vi "Drive Controller.vi"(8 "error in":errorcluster) -> ()   [LabVIEW 2016]
doc: "This VI executes continuously carrying out the current operation and responding to updates or new operation requests. It will often contain the timing or control code that is difficult to place directly in TeleOp. This VI generally opens all sensors and motors and isolates the rest of the robot code from knowing implementation details of how the operations are carried out."
uses:
  Drive Setpoints.ctl
  Drive Operations.ctl
  <vilib>/Rock Robotics/WPI/SafetyOutput/WPI_SafetyOutputConfigMenu.ctl
  <vilib>/Rock Robotics/SystemInterfaces/DIO/FPGA_DIOPWMChannel.ctl
  Utility/Drive for Distance States.ctl
  <vilib>/Rock Robotics/WPI/RobotDrive/WPI_RobotDriveOpen4MotorWithTalon.vi
panel:
  out "Setpoints":T1(graph)
  out "Current\nCmd":string
  # "Tip: It may be helpful to observe inputs and sensor values.\nYou may also want to display tuning or debugging controls."
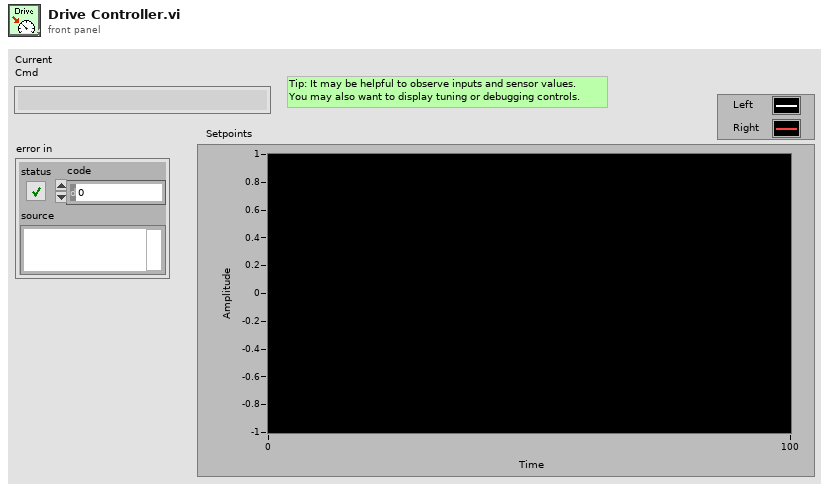
[diagram p1: front panel]
types:
  T1 = cluster{"Left Setpoint":dbl, "Right Setpoint":dbl}
  T2 = typedef "FPGA_DIOPWMChannel.ctl" = enum8{"PWM 0", "PWM 1", "PWM 2", "PWM 3", "PWM 4", "PWM 5", "PWM 6", "PWM 7", "PWM 8", "PWM 9", "PWM MXP 0", "PWM MXP 1", "PWM MXP 2", "PWM MXP 3", "PWM MXP 4", "PWM MXP 5", "PWM MXP 6", "PWM MXP 7", "PWM MXP 8", "PWM MXP 9", "Invalid"}
  T3 = typedef "WPI_SafetyOutputConfigMenu.ctl" = enum16{"Enable", "Disable"}
  T4 = typedef "Drive Setpoints.ctl" = cluster{"Operation":T5, "Left Setpoint":dbl, "Right Setpoint":dbl, "Duration":dbl, "Distance":dbl, "Degrees Rotation":dbl, "Clockwise?":bool}
  T5 = typedef "Drive Operations.ctl" = enum16{"Reserve", "Read Current", "Immediate", "Drive for Time", "Drive for Distance", "Rotate"}
  T6 = typedef "WPI_RobotDriveDevRef.ctl" = cluster{"DevStatus":errorcluster, "Motors[]":T7[], "Square Inputs":bool, "Max Output":dbl}
  T7 = typedef "WPI_MotorControlDeviceRef.ctl" = cluster{"DeviceStatus":errorcluster, "Type":T8, "PWM":cluster{"PWM Channel":T2, "DeadBand":T9}, "CAN":cluster{"Device Number":u8, "SetOutput VI Ref":variant, "GetOutput VI Ref":variant, "Enable VI Ref":variant, "Disable VI Ref":variant, "Data":variant}, "Invert":bool}
  T8 = typedef "WPI_MotorControlType.ctl" = enum16{"PWM", "CAN"}
  T9 = typedef "WPI_PWMDeadband.ctl" = cluster{"Name":string, "maxPositivePwm":i32, "minPositivePwm":i32, "centerPwm":i32, "maxNegativePwm":i32, "minNegativePwm":i32, "angularRange":u16}
  T10 = typedef "Command Status Info.ctl" = cluster{"Name":string, "Status":T11, "notifier out":T12}
  T11 = typedef "Completion Status.ctl" = enum16{"Successful", "Aborted", "Incomplete"}
  T12 = typedef "Completion Notifier.ctl" = refnum<notifier>
  T13 = cluster{"SubSystem Data":T4, cluster{"Start Time (ms)":u32, "Iterations":i32}, cluster{"Command Info":T10, "Description":string, "SubSystem Data":T4, "notifier out":refnum<notifier>, "Subsystem Name":string}}
  T14 = typedef "Drive for Distance States.ctl" = enum16{"Check Distance", "Initialize Distance"}
  T15 = cluster{"SubSystem Data":T4, cluster{"Start Time (ms)":u32, "Iterations":i32}, "Default Command Arguments":cluster{"Command Info":T10, "Description":string, "SubSystem Data":T4, "notifier out":refnum<notifier>, "Subsystem Name":string}}
  T16 = cluster{"Don't move motors while reserved":dbl, "Don't move motors while reserved":dbl}
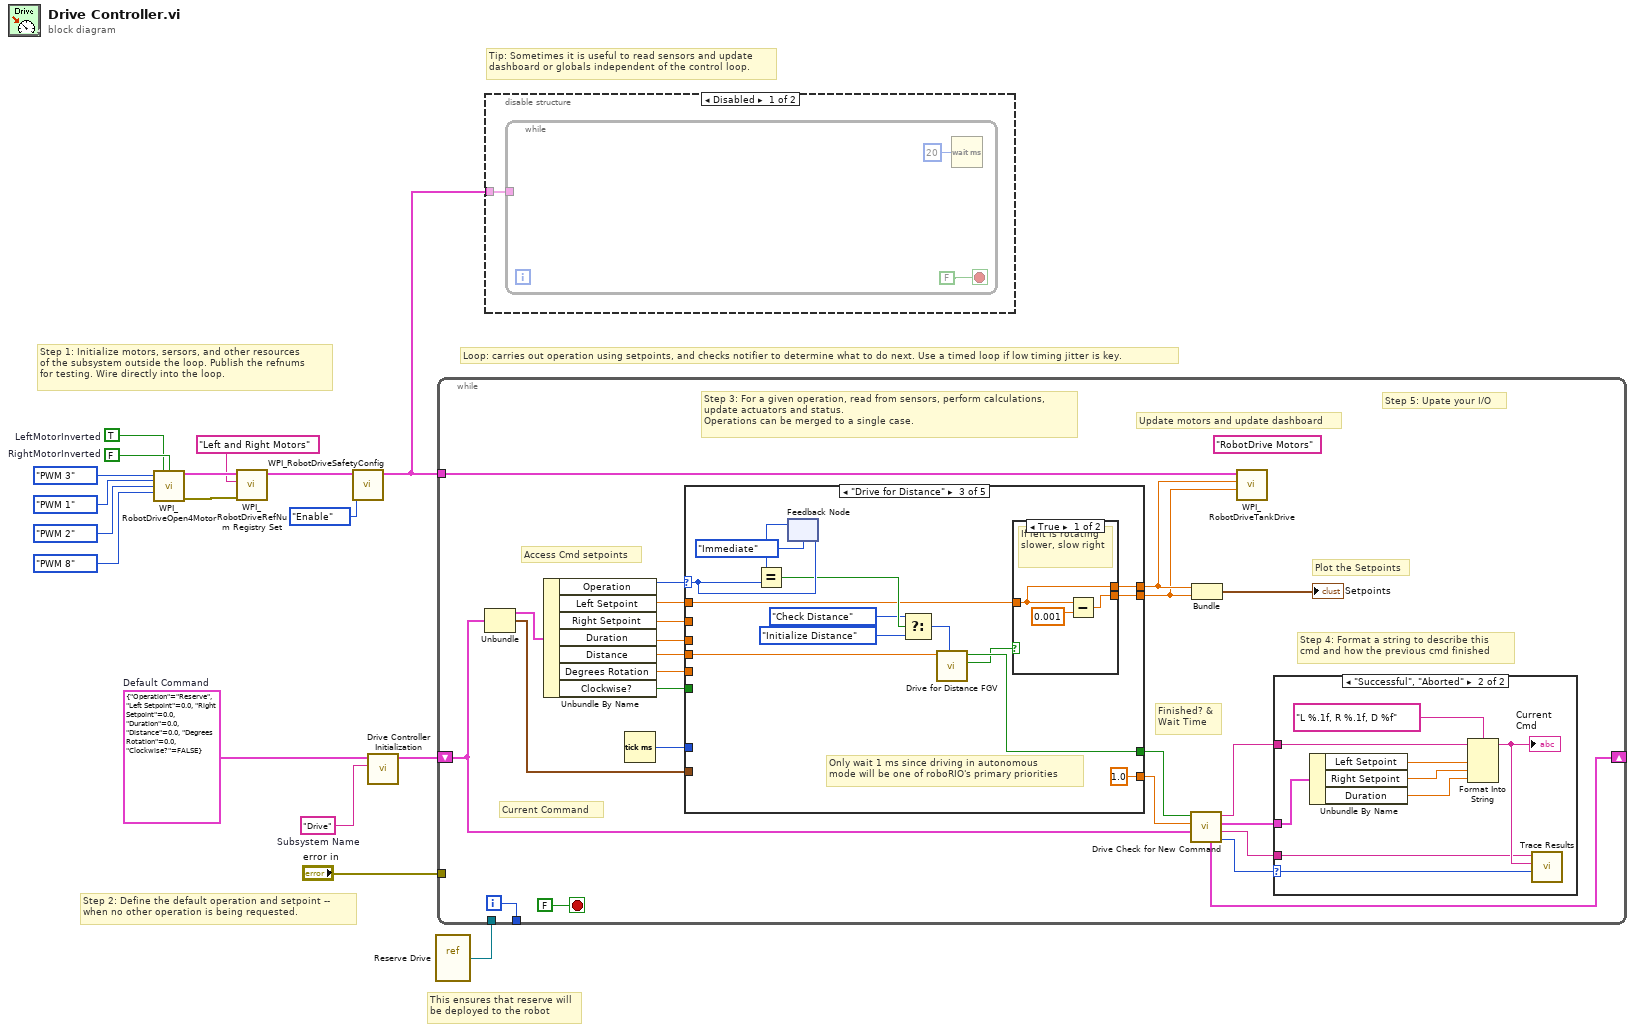
[diagram p0: block diagram]
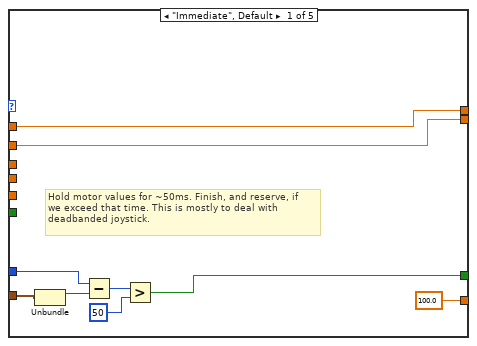
[diagram p4: hidden frame]
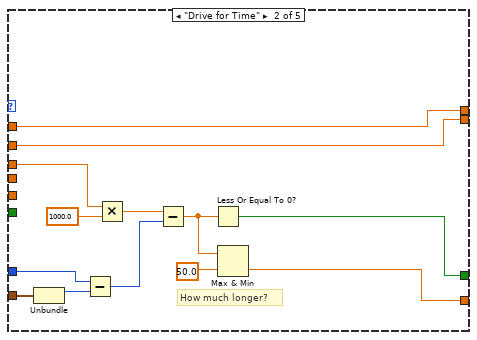
[diagram p5: hidden frame]
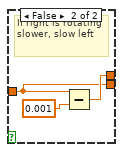
[diagram p6: hidden frame]
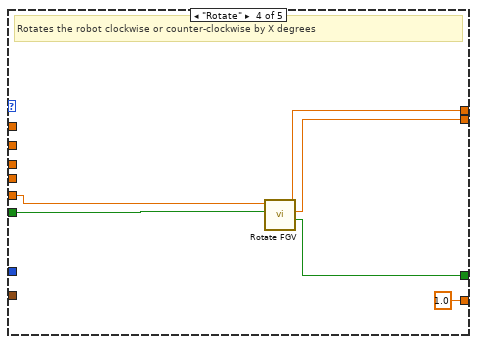
[diagram p7: hidden frame]
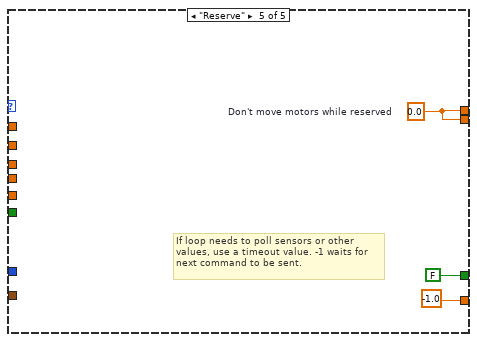
[diagram p8: hidden frame]
diagram:
  w14 = TRUE  # LeftMotorInverted
  w15 = FALSE  # RightMotorInverted
  w16 = T4 {"Operation"=enum."Reserve", "Left Setpoint"=0.0, "Right Setpoint"=0.0, "Duration"=0.0, "Distance"=0.0, "Degrees Rotation"=0.0, "Clockwise?"=FALSE}  # Default Command
  w17 = "Drive"  # Subsystem Name
  # "This ensures that reserve will\nbe deployed to the robot"
  # "Tip: Sometimes it is useful to read sensors and update\ndashboard or globals independent of the control loop."
  # "Step 2: Define the default operation and setpoint --\nwhen no other operation is being requested."
  # "Step 1: Initialize motors, sersors, and other resources\nof the subsystem outside the loop. Publish the refnums\nfor testing. Wire directly into the loop."
  # "Loop: carries out operation using setpoints, and checks notifier to determine what to do next. Use a timed loop if low timing jitter is key."
  n1 = call-poly <vilib>:"WPI_RobotDriveOpen4Motor.vi"("Rear Left Motor"=FPGA_DIOPWMChannel."PWM 3", "Rear Left Motor Inverted"=w14, "Rear Right Motor Inverted"=w15, "Rear Right Motor"=FPGA_DIOPWMChannel."PWM 1" ("Rear Left Motor"), "Front Left Motor"=FPGA_DIOPWMChannel."PWM 2" ("Rear Left Motor"), "Front Right Motor"=FPGA_DIOPWMChannel."PWM 8" ("Rear Left Motor")) -> ("RobotDriveDevRef"=w13:T6, "error out"=w11:errorcluster)  [unwired: 8 in]
  n2 = call <vilib>:"WPI_RobotDriveRefNum Registry Set.vi"("error in (no error)"=w11, "refnum name"="Left and Right Motors", "RobotDriveDevRef"=w13) -> ("RobotDriveDevRef"=w10:T6)  [unwired: 1 in, 7 out]
  n3 = call <vilib>:"WPI_RobotDriveSafetyConfig.vi"("mode"=WPI_SafetyOutputConfigMenu."Enable", "RobotDriveDevRef"=w10) -> ("RobotDriveDevRef"=w8:T6)  [unwired: 8 in, 1 out]
  n4 = call "Drive Controller Initialization.vi"("Subsystem Name"=w17, "Default Command"=w16) -> ("output cluster"=w6:T13)  [unwired: 9 in]
  n5 = vi-ref "Reserve Drive.vi"() -> (w5:refnum<vi>)
  n6 = while {
    shift-right: [w28] -> _
    shift-left: w6 -> [w21]
    tunnel: [w40] -> _
    tunnel: w8 -> [w36]
    tunnel: "error in" -> [_]
    tunnel: w5 -> [_]
    i -> [w40]
    stop <- FALSE stop-if-true
    (unwired) "RobotDrive Motors" ("Name")
    # "Step 5: Upate your I/O"
    # "Step 4: Format a string to describe this\ncmd and how the previous cmd finished"
    # "Current Command"
    # "Update motors and update dashboard"
    # "Plot the Setpoints"
    # "Access Cmd setpoints"
    # "Finished? &\nWait Time"
    # "Step 3: For a given operation, read from sensors, perform calculations,\nupdate actuators and status.\nOperations can be merged to a single case."
    n7 = Unbundle(w21) -> ("SubSystem Data"=w35:T4, w22:cluster{"Start Time (ms)":u32, "Iterations":i32})  [unwired: 1 out]
    n8 = Unbundle By Name(w35) -> ("Operation"=w34:T5, "Left Setpoint"=w33:dbl, "Right Setpoint"=w32:dbl, "Duration"=w31:dbl, "Distance"=w20:dbl, "Degrees Rotation"=w19:dbl, "Clockwise?"=w18:bool)
    n9 = Tick Count (ms)() -> (millisecond timer value=w30:u32)
    n10 = case shown="\"Drive for Distance\"" w34 {
      selector: w34 -> [_ _ w85 _ _]
      tunnel: [100.0 w60 1.0 1.0 -1.0] -> w27
      tunnel: [w52 w67 w79 w94 FALSE ("ignore previous (F)")] -> w26
      tunnel: w22 -> [w51 w69 _ _ _]
      tunnel: [w58 w66 w75 w96 w99] -> w38
      tunnel: [w57 w65 w76 w95 w99] -> w37
      tunnel: w33 -> [w58 w66 w77 _ _]
      tunnel: w32 -> [w57 w65 _ _ _]
      tunnel: w31 -> [_ w64 _ _ _]
      tunnel: w30 -> [w53 w63 _ _ _]
      tunnel: w20 -> [_ _ w73 _ _]
      tunnel: w19 -> [_ _ _ w97 _]
      tunnel: w18 -> [_ _ _ w93 _]
      frame "Immediate", Default {
        # "Hold motor values for ~50ms. Finish, and reserve, if\nwe exceed that time. This is mostly to deal with\ndeadbanded joystick."
        n11 = Unbundle(w51) -> ("Start Time (ms)"=w54:u32)  [unwired: 1 out]
        n12 = Subtract(x=w53, y=w54) -> (x-y=w55:u32)
        n13 = Greater?(x=w55, y=u8 50 ("Left Motor")) -> (0:w52:bool)
      }
      frame "Drive for Time" {
        # "How much longer?"
        n14 = Unbundle(w69) -> ("Start Time (ms)"=w68:u32)  [unwired: 1 out]
        n15 = Subtract(x=w63, y=w68) -> (x-y=w72:u32)
        n16 = Multiply(x=w64, y=1000.0) -> (x*y=w71:dbl)
        n17 = Subtract(x=w71, y=w72) -> (x-y=w62:dbl)
        n18 = Less Or Equal To 0?(x=w62) -> (x <= 0?=w67:bool)
        n19 = Max & Min(x=w62, y=50.0) -> (min(x,y)=w60:dbl)  [unwired: 1 out]
      }
      frame "Drive for Distance" {
        # "Only wait 1 ms since driving in autonomous \nmode will be one of roboRIO's primary priorities"
        n20 = feedback-in #1(w85) -> ()
        n21 = feedback #1(Drive_Operations."Immediate" ("Operation")) -> (w86:T5)
        n22 = Equal?(x=w86, y=w85) -> (x = y?=w83:bool)
        n23 = Select(t=Drive_for_Distance_States."Check Distance" ("State"), s=w83, f=Drive_for_Distance_States."Initialize Distance" ("State")) -> (s? t:f=w80:T14)
        n24 = call "Drive for Distance FGV.vi"("State"=w80, "Desired Distance"=w73) -> ("Slow: Left (T) / Right (F)"=w78:bool, "Complete?"=w79:bool)  [unwired: 7 in, 1 out]
        n25 = case shown="True" w78 {
          tunnel: w77 -> [w87 w90]
          tunnel: [w88 w90] -> w76
          tunnel: [w87 w91] -> w75
          frame True {
            # "If left is rotating\nslower, slow right"
            n26 = Subtract(x=w87, y=0.001) -> (x-y=w88:dbl)
          }
          frame False {
            # "If right is rotating\nslower, slow left"
            n27 = Subtract(x=w90, y=0.001) -> (x-y=w91:dbl)
          }
        }
      }
      frame "Rotate" {
        # "Rotates the robot clockwise or counter-clockwise by X degrees"
        n28 = call "Rotate FGV.vi"("Clockwise?"=w93, "Degrees Rotation"=w97) -> ("Complete?"=w94:bool, "Right Setpoint"=w95:dbl, "Left Setpoint"=w96:dbl)  [unwired: 6 in, 1 out]
      }
      frame "Reserve" {
        w99 = 0.0  # Don't move motors while reserved
        # "If loop needs to poll sensors or other\nvalues, use a timeout value. -1 waits for\nnext command to be sent."
      }
    }
    n29 = call "Drive Check for New Command.vi"("input cluster"=w21, "Wait time (ms)"=w27, "Finished?"=w26) -> ("Completion"=w29:T11, "Subsystem Name"=w23:string, "SetPoint"=w24:T4, "Initial Trace String"=w25:string, "output cluster"=w28:T15)  [unwired: 4 in]
    n30 = Bundle("Don't move motors while reserved"=w38, "Don't move motors while reserved"=w37) -> (→"Setpoints":T16)  [unwired: 1 in]
    n31 = call <vilib>:"WPI_RobotDriveTankDrive.vi"("Right axis value"=w37, "Left axis value"=w38, "RobotDriveDevRef"=w36) -> ()  [unwired: 6 in, 3 out]
    n32 = case shown="\"Successful\", \"Aborted\"" w29 {
      selector: w29 -> [_ w50]
      tunnel: w25 -> [_ w45]
      tunnel: w24 -> [_ w46]
      tunnel: w23 -> [_ w42]
      frame "Incomplete", Default {
        # "Continuing current command"
      }
      frame "Successful", "Aborted" {
        # "Report and setup for next command"
        n33 = Unbundle By Name(w46) -> ("Left Setpoint"=w48:dbl, "Right Setpoint"=w49:dbl, "Duration"=w43:dbl)
        n34 = Format Into String(format string="L %.1f, R %.1f, D %f", initial string=w45, w48, w49, w43) -> (resulting string=w44:string)  [unwired: 1 in, 1 out]
        "Current\nCmd" <- w44
        n35 = call <vilib>:"Trace Results.vi"("Status of previous command"=w50, "Description"=w44, "Subsystem"=w42) -> ()  [unwired: 9 in]
      }
    }
  }
  n36 = disable-structure shown="Disabled" {
    disable-tunnel: w8 -> [w102 _]
    frame Disabled {
      n37 = while {
        tunnel: w102 -> [_]
        stop <- FALSE stop-if-true
        n38 = Wait (ms)(milliseconds to wait=u32 20) -> ()  [unwired: 1 out]
      }
    }
    frame Enabled {
    }
  }
